vi "Create-and-send-heartbeat.vi"(6 "Timeout":i32=-1, 8 "error in (no error)":errorcluster, 9 "Sender ID":i32, 10 "Sender":string, 11 "Server channel":refnum<queue>) -> (0 "error out":errorcluster)   [LabVIEW 2013, in "Messages.lvlib" / "Heartbeat.lvclass"]
uses:
  Heartbeat.lvclass
  Message.lvclass
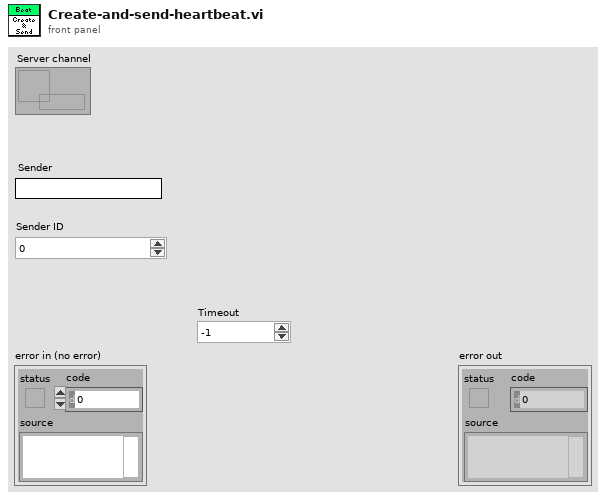
[diagram p1: front panel]
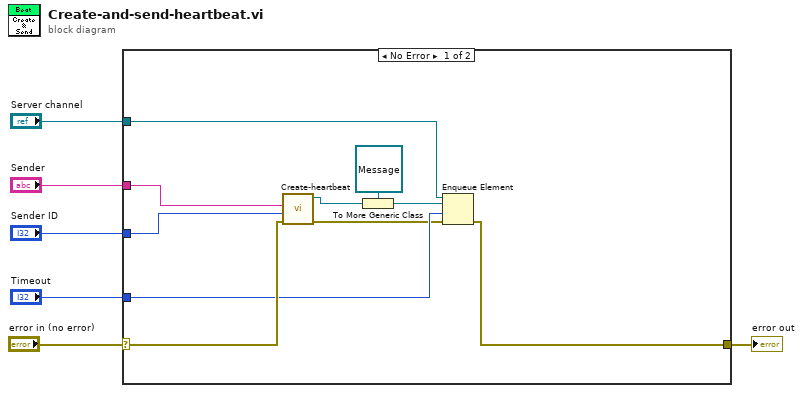
[diagram p0: block diagram]
diagram:
  n1 = case shown="No Error" "error in (no error)" {
    selector: "error in (no error)" -> [w13 w17]
    tunnel: [w7 w17] -> w5
    tunnel: "Sender" -> [w16 _]
    tunnel: "Sender ID" -> [w15 _]
    tunnel: "Server channel" -> [w14 _]
    tunnel: "Timeout" -> [w12 _]
    frame No Error {
      n2 = call "Create-heartbeat.vi"("error in (no error)"=w13, "Sender ID"=w15, "Sender"=w16) -> ("error out"=w11:errorcluster, "Heartbeat out"=w10:refnum<class "Heartbeat.lvclass">)  [unwired: 7 in]
      n3 = To More Generic Class(target class=refnum<class "Message.lvclass"> refnum ("Messages.lvlib:Message.lvclass"), reference=w10) -> (generic class reference=w9:refnum<class "Message.lvclass">)
      n4 = Enqueue Element(queue=w14, element=w9, timeout in ms (-1)=w12, error in (no error)=w11) -> (error out=w7:errorcluster)  [unwired: 2 out]
    }
    frame Error {
    }
  }
  "error out" <- w5
